vi "Digital Write Multiple.vi"(8 "error in (no error)":errorcluster, 10 "Digital Data":bool[](array[boolean]), 11 "Digital Writer in":refnum<class "Digital Writer.lvclass">) -> (0 "error out":errorcluster, 3 "Digital Writer out":refnum<class "Digital Writer.lvclass">)   [LabVIEW 2024, in "DAQmx Actor.lvlib" / "Digital Writer.lvclass"]
uses:
  Digital Writer.lvclass
  Digital Writer.lvclass/Digital Writer.ctl
  <vilib>/DAQmx/write.llb/DAQmx Write (Digital 1D Bool NChan 1Samp 1Line).vi
  <vilib>/DAQmx/miscellaneous.llb/DAQmx Fill In Error Info.vi
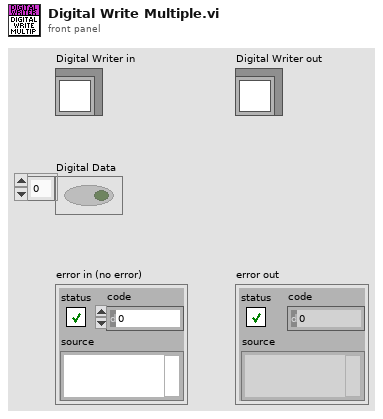
[diagram p1: front panel]
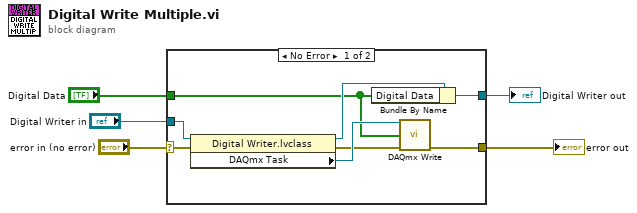
[diagram p0: block diagram]
diagram:
  n1 = case shown="No Error" "error in (no error)" {
    selector: "error in (no error)" -> [w12 w15]
    tunnel: [w9 w15] -> w4
    tunnel: [w6 w14] -> w2
    tunnel: "Digital Writer in" -> [w13 w14]
    tunnel: "Digital Data" -> [w7 _]
    frame No Error {
      n2 = property class="Digital Writer.lvclass"(reference=w13, error in=w12) -> (reference out=w8:refnum<class "Digital Writer.lvclass">, error out=w10:errorcluster, "DAQmx Task"=w11:refnum<k21>)
      n3 = Bundle By Name(cluster=w8, "Digital Data"=w7) -> (w6:refnum<class "Digital Writer.lvclass">)
      n4 = call-poly <vilib>:"DAQmx Write.vi"("task/channels in"=w11, "data"=w7, "error in"=w10) -> ("error out"=w9:errorcluster)  [unwired: 10 in, 2 out]
    }
    frame Error {
    }
  }
  "error out" <- w4
  "Digital Writer out" <- w2
